vi "Database Recordset Move.vi"(8 "error in (no error)":errorcluster caption="错误输入（无错误）", 9 "NumRecords":i32, 11 "Database Recordset 输入":refnum<class "Database Recordset.lvclass"> caption="DNL_LabVIEW Object in") -> (0 "error out":errorcluster caption="错误输出", 3 "Database Recordset 输出":refnum<class "Database Recordset.lvclass"> caption="DNL_LabVIEW Object out")   [LabVIEW 2011, in "Database Recordset.lvclass"]
uses:
  Database Recordset.lvclass
  Database Recordset.lvclass/Database Recordset.ctl
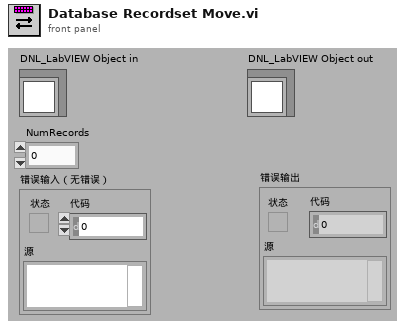
[diagram p1: front panel]
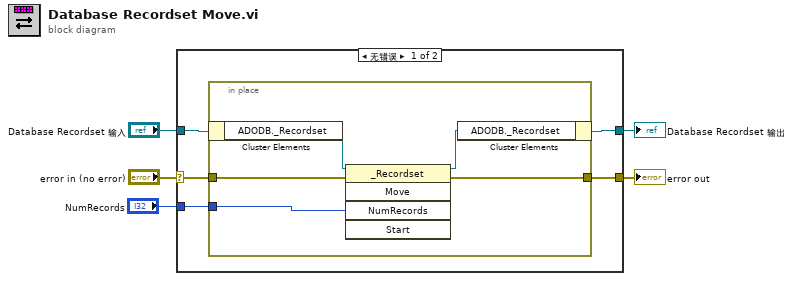
[diagram p0: block diagram]
diagram:
  n1 = case shown="无错误" "error in (no error)" {
    selector: "error in (no error)" -> [w8 w17]
    tunnel: [w7 w17] -> w4
    tunnel: [w9 w16] -> w2
    tunnel: "Database Recordset 输入" -> [w10 w16]
    tunnel: "NumRecords" -> [w6 _]
    frame No Error {
      n2 = in-place {
        in-place-border: w8 -> [w13]
        in-place-border: [w12] -> w7
        in-place-border: w6 -> [w11]
        n3 = in-place-cluster #1(w10) -> ("ADODB._Recordset"=w15:refnum<k7>)
        n4 = invoke class="_Recordset" method="Move"(reference=w15, error in=w13, "NumRecords"=w11) -> (reference out=w14:refnum<k7>, error out=w12:errorcluster)  [unwired: 2 in, 3 out]
        n5 = in-place-cluster #1("ADODB._Recordset"=w14) -> (w9:refnum<class "Database Recordset.lvclass">)
      }
    }
    frame Error {
    }
  }
  "error out" <- w4
  "Database Recordset 输出" <- w2
